vi "Read Send Builder.vi"(11 "Message Scripter in":refnum<class "Message Scripter.lvclass">) -> (2 "Send Builder":refnum<class "Send Builder.lvclass">)   [LabVIEW 2020, in "Message Maker.lvlib" / "Message Scripter.lvclass"]
uses:
  Message Scripter.lvclass
  Send Builder/Send Builder.lvclass
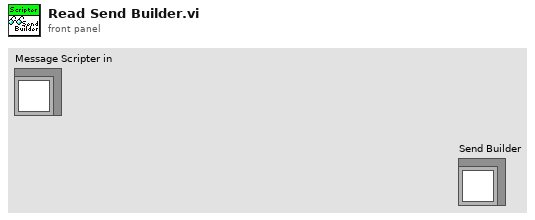
[diagram p1: front panel]
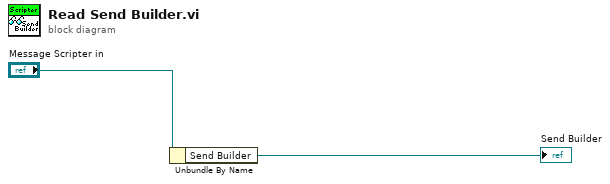
[diagram p0: block diagram]
diagram:
  n1 = Unbundle By Name("Message Scripter in") -> ("Send Builder"=→"Send Builder":refnum<class "Send Builder.lvclass">)
